vi "test Get Channel Version.vi"(11 "Test Case In":refnum<class "Test PCANBasic.lvclass">) -> (0 "error out":errorcluster, 3 "Test Case Out":refnum<class "Test PCANBasic.lvclass">)   [LabVIEW 2020, in "Test PCANBasic.lvclass"]
uses:
  Test PCANBasic.lvclass
  C:/Program Files/National Instruments/LabVIEW 2025/vi.lib/Astemes/LUnit/Test Case.lvclass
  <vilib>/Astemes/LUnit/Test Case.lvclass/Test Case.ctl
  Test PCANBasic.lvclass/Test PCANBasic.ctl
  <vilib>/Astemes/LUnit/Test Case.lvclass
  Global PCAN Channel.vi
  source/PCANBasic.lvlib
  C:/Program Files/National Instruments/LabVIEW 2025/vi.lib/Astemes/LUnit/LUnit Runnable.lvclass
  D:/git/PCAN-Basic-LabVIEW/tests/Tests PCANBasic/Test PCANBasic.lvclass
panel:
  out "Channel Version":string
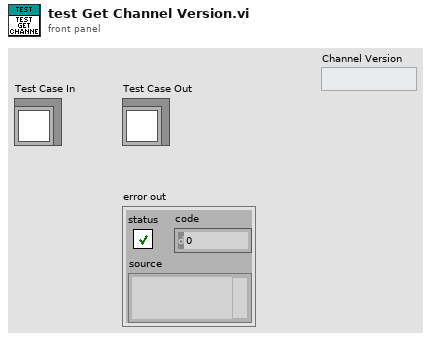
[diagram p1: front panel]
types:
  T1 = typedef "PCANBasic.lvlib/TPCANHandle.ctl" = u16
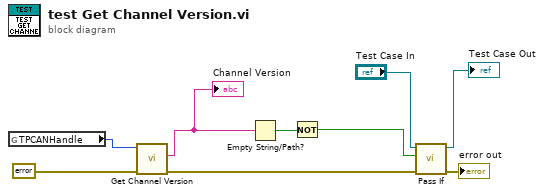
[diagram p0: block diagram]
diagram:
  n1 = global read "Global PCAN Channel.vi" "TPCANHandle"() -> (w4:T1)
  n2 = call "Get Channel Version.vi"("error in"=errorcluster {"status"=FALSE, "code"=0, "source"=""}, "TPCANHandle in"=w4) -> ("error out"=w5:errorcluster, "Channel Version"=w1:string)  [unwired: 6 in, 2 out]
  "Channel Version" <- w1
  n3 = Empty String/Path?(string/path=w1) -> (empty?=w3:bool)
  n4 = Not(x=w3) -> (.not. x?=w2:bool)
  n5 = call <vilib>:"Pass If.vi"("error in (no error)"=w5, "Pass?"=w2, "LUnit Test Case In"="Test Case In") -> ("error out"=→"error out":errorcluster, "LUnit Test Case Out"=→"Test Case Out":refnum<class "Test PCANBasic.lvclass">)  [unwired: 7 in]
